vi "pockelscellcalibration.vi"(1 "l":dbl, 2 "T":dbl) -> (0 "Vout":dbl)   [LabVIEW 2015]
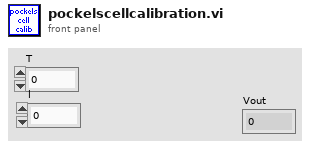
[diagram p1: front panel]
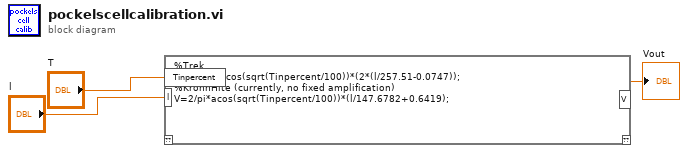
[diagram p0: block diagram]
diagram:
  n1 = script code="%Trek\n%V=2/pi*acos(sqrt(Tinpercent/100))*(2*(l/257.51-0.0747)); \n%KrohnHite (currently, no fixed amplification)\nV=2/pi*acos(sqrt(Tinpercent/100))*(l/147.6782+0.6419);"("Tinpercent"="T", "l"="l") -> ("V"=→"Vout":dbl)  [unwired: 1 in, 1 out]
